vi "RobotMain.vi"() -> ()   [LabVIEW 2014]
uses:
  Command.ctl
  DataHighway.ctl
  <vilib>/vision/Image Controls.llb/IMAQ Image.ctl
  <vilib>/myRIO/Common/Instrument Driver Framework/myRIO v1.0/UART/vis/myRIO v1.0 Close UART.vi
  <vilib>/myRIO/Common/Instrument Driver Framework/Utilities/vis/FPGA Ref Manager.vi
  <vilib>/myRIO/Common/Instrument Driver Framework/myRIO v1.0/myRIO v1.0 Reset FPGA.vi
  <vilib>/myRIO/Common/Instrument Driver Framework/myRIO v1.0/IRQ/vis/myRIO v1.0 IRQ Info FGV.vi
  <vilib>/myRIO/Common/Instrument Driver Framework/myRIO v1.0/IRQ/vis/myRIO v1.0 Timer IRQ Info FGV.vi
  <vilib>/myRIO/Common/Instrument Driver Framework/myRIO v1.0/IRQ/vis/myRIO v1.0 ISR Agent.vi
  <vilib>/ErrorRing/Error Ring.xnode
  <vilib>/myRIO/Instrument Drivers/Utilities/Utilities.lvlib
panel:
  out "DataHWay":T1
  out "ComHWayFromOCU":T3 {"Pan" scale=-2.0..10.0; "Tilt" scale=-10.0..10.0}
  in  "stop robot control":bool
  out "error out":errorcluster
  # "Robot will run headless\nwithout a control panel\nso keep this control panel\nas simple as possible while\nstill allowing debugging."
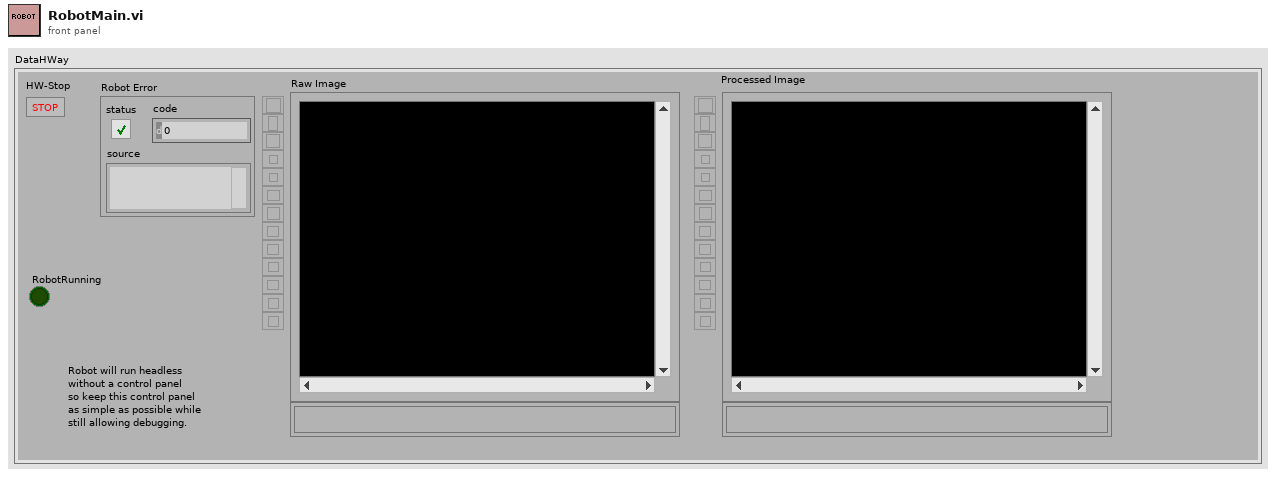
[diagram p1: front panel]
types:
  T1 = typedef "DataHighway.ctl" = cluster{"HW-Stop":bool, "RobotRunning":bool, "Robot Error":errorcluster, "Raw Image":T2, "Processed Image":T2}
  T2 = typedef "IMAQ Image.ctl" = refnum<image>
  T3 = typedef "Command.ctl" = cluster{"States":enum16{"Initialize", "Wait for Event", "Debug Robot", "Run Robot", "Exit"}, "E-Stop":bool, "Tilt":dbl, "Pan":dbl}
  T4 = enum16{"Initialize", "Wait for Event", "Debug Robot", "Run Robot", "Exit"}
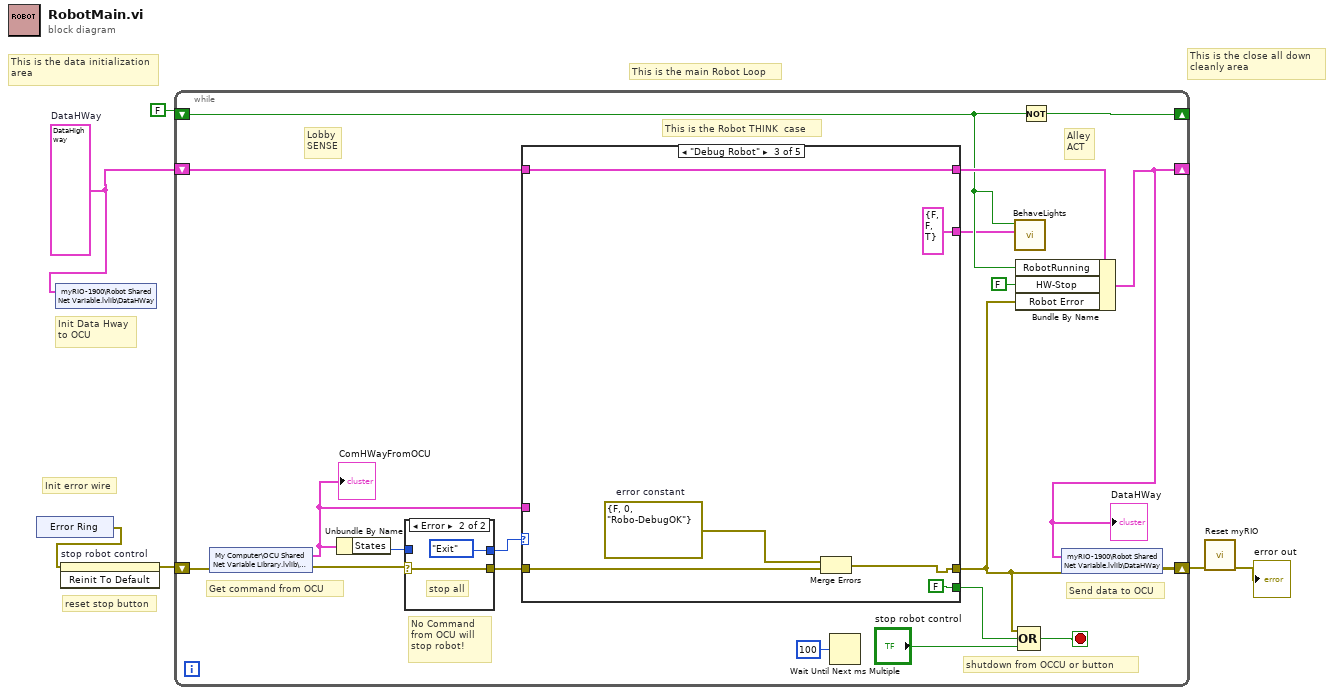
[diagram p0: block diagram]
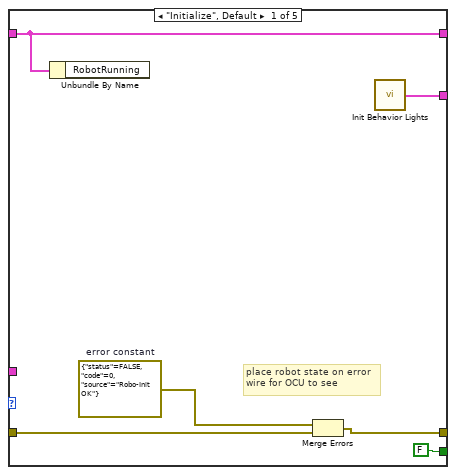
[diagram p3: hidden frame]
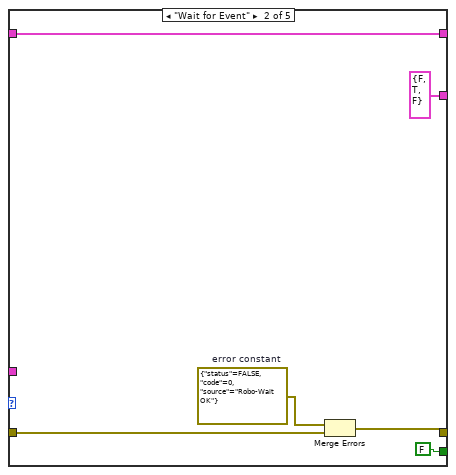
[diagram p4: hidden frame]
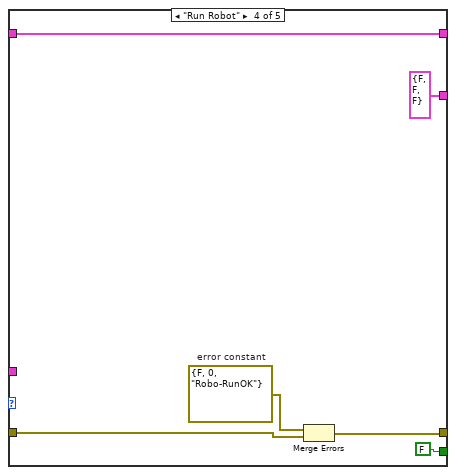
[diagram p5: hidden frame]
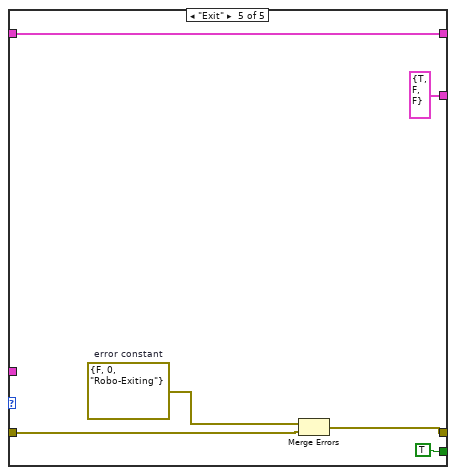
[diagram p6: hidden frame]
diagram:
  w3 = T1 {"HW-Stop"=FALSE, "RobotRunning"=FALSE, "Robot Error"={"status"=FALSE, "code"=0, "source"=""}, "Raw Image"=refnum, "Processed Image"=refnum}  # DataHWay
  # "reset stop button"
  # "Init error wire"
  # "Init Data Hway\nto OCU"
  # "This is the close all down \ncleanly area"
  # "This is the data initialization\narea"
  # "This is the main Robot Loop"
  n1 = xnode "Error Ring"() -> ("error out"=w2:errorcluster)
  n2 = shared-variable "myRIO-1900\\Robot Shared Net Variable.lvlib\\DataHWay"(w3) -> ()  [unwired: 1 in, 1 out]
  n3 = invoke on="stop robot control" class="Bool" method="Reinit To Default"(error in=w2) -> (error out=w1:errorcluster)  [unwired: 2 in, 2 out]
  n4 = while {
    shift-right: [w16] -> w5
    shift-left: w1 -> [w13]
    shift-right: [w11] -> _
    shift-left: w3 -> [w20]
    shift-right: [w15] -> _
    shift-left: FALSE -> [w9]
    stop <- w23 stop-if-true
    # "No Command \nfrom OCU will\nstop robot!"
    # "Get command from OCU"
    # "Send data to OCU"
    # "shutdown from OCCU or button"
    # "Alley\nACT"
    # "This is the Robot THINK  case"
    # "Lobby\nSENSE"
    n5 = shared-variable "My Computer\\OCU Shared Net Variable Library.lvlib\\ComHWay"(error in=w13) -> (w17:T3, error out=w12:errorcluster)
    "ComHWayFromOCU" <- w17
    n6 = Unbundle By Name(w17) -> ("States"=w18:T4)
    n7 = case shown="Error" w12 {
      selector: w12 -> [w27 w29]
      tunnel: [w27 w29] -> w24
      tunnel: [w26 T4."Exit" ("States")] -> w25
      tunnel: w18 -> [w26 _]
      frame No Error {
      }
      frame Error {
        # "stop all"
      }
    }
    n8 = case shown="\"Debug Robot\"" w25 {
      tunnel: w24 -> [w34 w39 w45 w51 w57]
      tunnel: [w33 w38 w44 w50 w56] -> w7
      tunnel: [FALSE FALSE FALSE FALSE TRUE] -> w22
      tunnel: w20 -> [w31 w40 w47 w53 w58]
      tunnel: [w31 w40 w47 w53 w58] -> w14
      tunnel: w17 -> [_ _ _ _ _]
      tunnel: [w30 cluster{"Red":bool, "Blue":bool, "Green":bool} {"Red"=FALSE, "Blue"=TRUE, "Green"=FALSE} ("Lights Out") cluster{"Red":bool, "Blue":bool, "Green":bool} {"Red"=FALSE, "Blue"=FALSE, "Green"=TRUE} ("Lights Out") cluster{"Red":bool, "Blue":bool, "Green":bool} {"Red"=FALSE, "Blue"=FALSE, "Green"=FALSE} ("Lights Out") cluster{"Red":bool, "Blue":bool, "Green":bool} {"Red"=TRUE, "Blue"=FALSE, "Green"=FALSE} ("Lights Out")] -> w8
      frame "Initialize", Default {
        w32 = errorcluster {"status"=FALSE, "code"=0, "source"="Robo-Init OK"}  # error constant
        # "place robot state on error\nwire for OCU to see"
        n9 = Unbundle By Name "Unbundle By Name"(w31) -> ()  [unwired: 1 out]
        n10 = Merge Errors "Merge Errors"(w32, w34) -> (w33:errorcluster)
        n11 = call "Init Behavior Lights.vi"() -> ("Lights Out"=w30:cluster{"Red":bool, "Blue":bool, "Green":bool})  [unwired: 11 in]
      }
      frame "Wait for Event" {
        w37 = errorcluster {"status"=FALSE, "code"=0, "source"="Robo-Wait OK"}  # error constant
        n12 = Merge Errors "Merge Errors"(w37, w39) -> (w38:errorcluster)
      }
      frame "Debug Robot" {
        w43 = errorcluster {"status"=FALSE, "code"=0, "source"="Robo-DebugOK"}  # error constant
        n13 = Merge Errors "Merge Errors"(w43, w45) -> (w44:errorcluster)
      }
      frame "Run Robot" {
        w49 = errorcluster {"status"=FALSE, "code"=0, "source"="Robo-RunOK"}  # error constant
        n14 = Merge Errors "Merge Errors"(w49, w51) -> (w50:errorcluster)
      }
      frame "Exit" {
        w55 = errorcluster {"status"=FALSE, "code"=0, "source"="Robo-Exiting"}  # error constant
        n15 = Merge Errors "Merge Errors"(w55, w57) -> (w56:errorcluster)
      }
    }
    n16 = Wait Until Next ms Multiple(millisecond multiple=u32 100) -> ()  [unwired: 1 out]
    n17 = call "BehaveLights.vi"("BehLightIn"=w8, "Blink"=w9) -> ()  [unwired: 9 in, 1 out]
    n18 = Bundle By Name(cluster=w14, "RobotRunning"=w9, "HW-Stop"=FALSE, "Robot Error"=w7) -> (w11:T1)
    "DataHWay" <- w11
    n19 = Compound Arithmetic op=OR(w7, w22, "stop robot control") -> (w23:bool)
    n20 = Not(x=w9) -> (.not. x?=w15:bool)
    n21 = shared-variable "myRIO-1900\\Robot Shared Net Variable.lvlib\\DataHWay"(w11, error in=w7) -> (error out=w16:errorcluster)
  }
  n22 = call <vilib>:"Reset myRIO.vi"("error in (no error)"=w5) -> ("error out"=→"error out":errorcluster)  [unwired: 10 in]
